vi "Read_Write_Trav_position.vi"(2 "Matched Configurations In":T1[](array[typedef]) {"Static Drive Configuration"."Indexer Mode  (FSA)" items=["Incremental", "Absolute"]; "Static Drive Configuration"."Buffer at Stop (SSH)" items=["Clear buffer", "Save and Continue"]; "Static Drive Configuration"."Buffer at Limit (SSG)" items=["Clear buffer", "Save and Continue"]; "Static Drive Configuration"."RS232 Echo Control (SSA)" items=["Echo ON", "Echo OFF"]; "Static Drive Configuration"."Reference edge of Home (OSH)" items=["CW", "CCW"]; "Static Drive Configuration"."Encoder Z for Home (OSD)" items=["Don't use", "Enable"]; "Static Drive Configuration"."Home Switch Sense (OSC)" items=["Normally Open", "Normally Closed"]; "Static Drive Configuration"."Home Position (OSB)" items=["Anywhere in Switch", "Edge of Switch"]; "Static Drive Configuration"."Limit Switch Sense (OSA)" items=["Normally Closed", "Normally Open"]; "Static Drive Configuration"."Limit Disable (LD)" items=["Both Enabled", "CW Disabled", "CCW Disabled", "Both Disabled"]; "Static Drive Configuration"."Stall Detect (FSH)" items=["Disable", "Enable"]; "Static Drive Configuration"."OP2 in Deadband (FSG)" items=["Don't Use", "ACTIVATE"]; "Static Drive Configuration"."Stop on Trigger 3 (FSF)" items=["Ignore", "STOP!"]; "Static Drive Configuration"."Activate OP1 on stall (FSE)" items=["Do not Activate", "ACTIVATE!"]; "Static Drive Configuration"."Stop on Stall (FSD)" items=["Continue", "STOP"]; "Static Drive Configuration"."Position Maintenance (FSC)" items=["Disabled", "Enabled"]; "Static Drive Configuration"."Step Mode  (FSB)" items=["Motor", "Encoder"]; "Static Drive Configuration"."Encoder Resolution (ER)" min=1 max=50000; "Static Drive Configuration"."Dead Band Window (DW)" min=0 max=999999999; "Static Drive Configuration"."Dead Band (DB)" min=0 max=999999999; "Static Drive Configuration"."Correction Gain % (CG)" items=["n/a", "12.5", "25", "37.5", "50", "62.5", "75", "87.5", "100"]; "Channel Properties"."Current Pos" format="%.2f"; "Channel Properties"."Backlash/Eng units" format="%.2f"; "Channel Properties"."Pulses/rev" format="%.2f"; "Channel Properties"."Pos Tolerance" format="%.2f"; "Channel Properties"."Pulses/unit" format="%.2f"; "Channel Properties"."Acc. Min" format="%.2f"; "Channel Properties"."Acc. Max" format="%.2f"; "Channel Properties"."Vel. Min" format="%.2f"; "Channel Properties"."Vel. Max" format="%.2f"; "Channel Properties"."Acc. Default" format="%.2f"; "Channel Properties"."Vel. Default" format="%.2f"}, 3 "Mode":T4(ring), 4 "Traverse Name":string="EnFlo Tunnel") -> (0 "Matched Configurations Out":T1[](array[typedef]) {"Static Drive Configuration"."Indexer Mode  (FSA)" items=["Incremental", "Absolute"]; "Static Drive Configuration"."Buffer at Stop (SSH)" items=["Clear buffer", "Save and Continue"]; "Static Drive Configuration"."Buffer at Limit (SSG)" items=["Clear buffer", "Save and Continue"]; "Static Drive Configuration"."RS232 Echo Control (SSA)" items=["Echo ON", "Echo OFF"]; "Static Drive Configuration"."Reference edge of Home (OSH)" items=["CW", "CCW"]; "Static Drive Configuration"."Encoder Z for Home (OSD)" items=["Don't use", "Enable"]; "Static Drive Configuration"."Home Switch Sense (OSC)" items=["Normally Open", "Normally Closed"]; "Static Drive Configuration"."Home Position (OSB)" items=["Anywhere in Switch", "Edge of Switch"]; "Static Drive Configuration"."Limit Switch Sense (OSA)" items=["Normally Closed", "Normally Open"]; "Static Drive Configuration"."Limit Disable (LD)" items=["Both Enabled", "CW Disabled", "CCW Disabled", "Both Disabled"]; "Static Drive Configuration"."Stall Detect (FSH)" items=["Disable", "Enable"]; "Static Drive Configuration"."OP2 in Deadband (FSG)" items=["Don't Use", "ACTIVATE"]; "Static Drive Configuration"."Stop on Trigger 3 (FSF)" items=["Ignore", "STOP!"]; "Static Drive Configuration"."Activate OP1 on stall (FSE)" items=["Do not Activate", "ACTIVATE!"]; "Static Drive Configuration"."Stop on Stall (FSD)" items=["Continue", "STOP"]; "Static Drive Configuration"."Position Maintenance (FSC)" items=["Disabled", "Enabled"]; "Static Drive Configuration"."Step Mode  (FSB)" items=["Motor", "Encoder"]; "Static Drive Configuration"."Encoder Resolution (ER)" min=1 max=50000; "Static Drive Configuration"."Dead Band Window (DW)" min=0 max=999999999; "Static Drive Configuration"."Dead Band (DB)" min=0 max=999999999; "Static Drive Configuration"."Correction Gain % (CG)" items=["n/a", "12.5", "25", "37.5", "50", "62.5", "75", "87.5", "100"]; "Channel Properties"."Current Pos" format="%.2f"; "Channel Properties"."Backlash/Eng units" format="%.2f"; "Channel Properties"."Pulses/rev" format="%.2f"; "Channel Properties"."Pos Tolerance" format="%.2f"; "Channel Properties"."Pulses/unit" format="%.2f"; "Channel Properties"."Acc. Min" format="%.2f"; "Channel Properties"."Acc. Max" format="%.2f"; "Channel Properties"."Vel. Min" format="%.2f"; "Channel Properties"."Vel. Max" format="%.2f"; "Channel Properties"."Acc. Default" format="%.2f"; "Channel Properties"."Vel. Default" format="%.2f"})   [LabVIEW 2011]
uses:
  AxisConfigCluster.ctl
  DriveProperties.ctl
  DriveStaticConfig.ctl
  Anemometry/Anemometry Sub Vis/Globals/Constants_global.vi
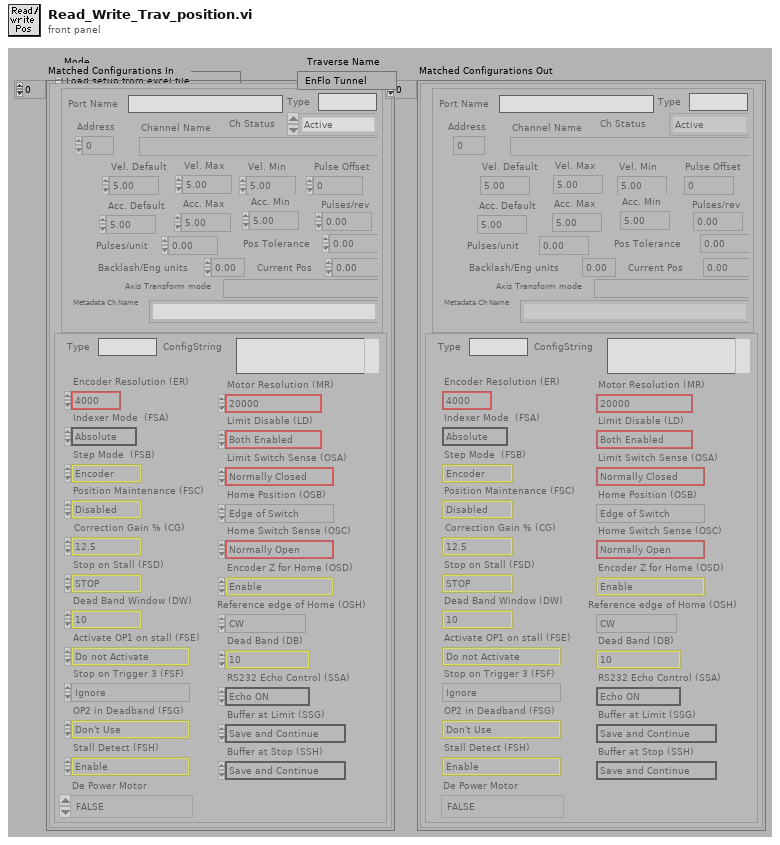
[diagram p1: front panel]
types:
  T1 = typedef "AxisConfigCluster.ctl" = cluster{"Channel Properties":T2, "Static Drive Configuration":T3}
  T2 = typedef "DriveProperties.ctl" = cluster{"Channel Name":string, "Vel. Default":dbl, "Acc. Default":dbl, "Vel. Max":dbl, "Vel. Min":dbl, "Acc. Max":dbl, "Acc. Min":dbl, "Pulses/unit":dbl, "Address":u8, "Pulse Offset":i32, "Pos Tolerance":dbl, "Pulses/rev":dbl, "Backlash/Eng units":dbl, "Current Pos":dbl, "Ch Status":enum16{"Active", "Offline", "Simulate"}, "Port Name":string, "Axis Transform mode":string, "Metadata Ch Name":string, "Type":string}
  T3 = typedef "DriveStaticConfig.ctl" = cluster{"Correction Gain % (CG)":u16, "Dead Band (DB)":i32, "Dead Band Window (DW)":i32, "Encoder Resolution (ER)":i32, "Step Mode  (FSB)":u16, "Position Maintenance (FSC)":u16, "Stop on Stall (FSD)":u16, "Activate OP1 on stall (FSE)":u16, "Stop on Trigger 3 (FSF)":u16, "OP2 in Deadband (FSG)":u16, "Stall Detect (FSH)":u16, "Limit Disable (LD)":u16, "Motor Resolution (MR)":enum16{"200", "400", "1000", "2000", "4000", "5000", "10000", "12800", "18000", "20000", "21600", "25000", "25400", "25600", "36000", "50000", "278528", "425984", "507904", "614400", "655360", "819200", "1024000"}, "Limit Switch Sense (OSA)":u16, "Home Position (OSB)":u16, "Home Switch Sense (OSC)":u16, "Encoder Z for Home (OSD)":u16, "Reference edge of Home (OSH)":u16, "RS232 Echo Control (SSA)":u16, "Buffer at Limit (SSG)":u16, "Buffer at Stop (SSH)":u16, "Indexer Mode  (FSA)":u16, "Type":string, "ConfigString":string, "De Power Motor":enum16{"TRUE", "FALSE"}}
  T4 = enum16{"Load setup from excel file", "Save setup to excel file"}
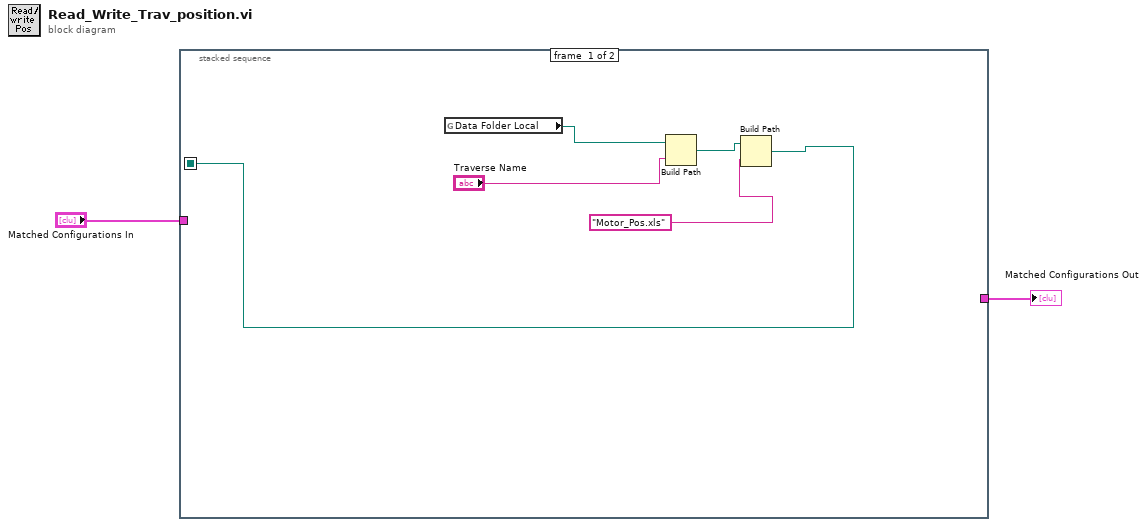
[diagram p0: block diagram]
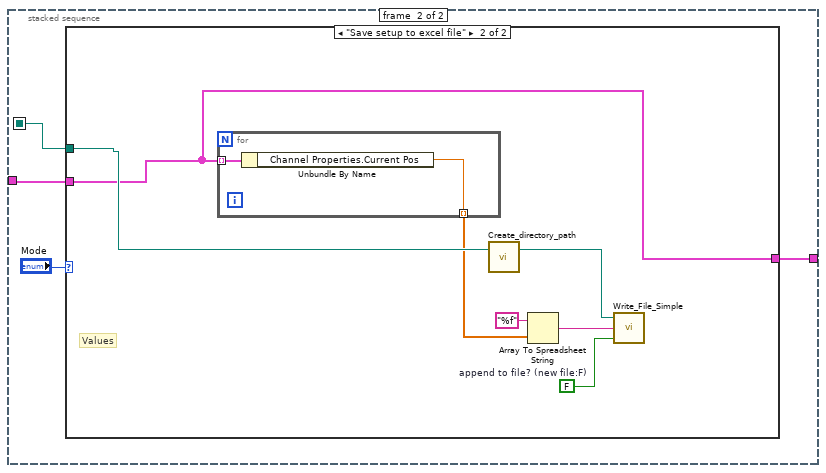
[diagram p2: hidden frame]
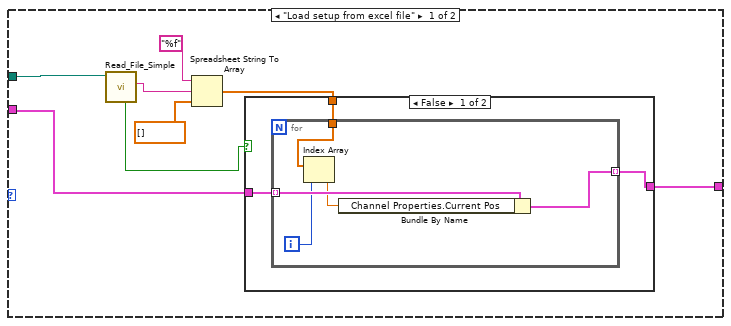
[diagram p3: hidden frame]
diagram:
  n1 = stacked-sequence {
    seq-local: [w4 _] -> [_ w10]
    tunnel: "Matched Configurations In" -> [_ w9]
    tunnel: [_ w8] -> w1
    frame #0 {
      n2 = global read "Constants_global.vi" "Data Folder Local"() -> (w5:path)
      n3 = Build Path(base path=w5, name or relative path="Traverse Name") -> (appended path=w3:path)
      n4 = Build Path(base path=w3, name or relative path="Motor_Pos.xls" ("Substring")) -> (appended path=w4:path)
    }
    frame #1 {
      n5 = case shown="\"Save setup to excel file\"" "Mode" {
        tunnel: w10 -> [w19 w31]
        tunnel: w9 -> [w18 w29]
        tunnel: [w17 w29] -> w8
        frame "Load setup from excel file" {
          n6 = call "Read_File_Simple.vi"("Filename"=w19) -> ("Error?"=w12:bool, "string"=w14:string)  [unwired: 2 in, 6 out]
          n7 = Spreadsheet String To Array(format string="%f", spreadsheet string=w14, array type (2D Dbl)=dbl[] []) -> (array=w13:dbl[])  [unwired: 1 out]
          n8 = case shown="False" w12 {
            tunnel: w18 -> [w22 w28]
            tunnel: [w21 w28] -> w17
            tunnel: w13 -> [w20 _]
            frame False {
              n9 = for {
                tunnel: w22 -> [w27] mode=indexing
                tunnel: [w26] -> w21 mode=indexing
                tunnel: w20 -> [w25]
                i -> [w24]
                n10 = Index Array(array=w25, index=w24) -> (element=w23:dbl)
                n11 = Bundle By Name(cluster=w27, "Channel Properties.Current Pos"=w23) -> (w26:T1)
              }
            }
            frame True {
            }
          }
        }
        frame "Save setup to excel file" {
          w33 = FALSE  # append to file? (new file:F)
          # "Values"
          n12 = for {
            tunnel: w29 -> [w37] mode=indexing
            tunnel: [w36] -> w30 mode=indexing
            n13 = Unbundle By Name(w37) -> ("Channel Properties.Current Pos"=w36:dbl)
          }
          n14 = call "Create_directory_path.vi"("Path name"=w31) -> ("Path name Out"=w35:path)  [unwired: 1 in, 1 out]
          n15 = Array To Spreadsheet String(array=w30, 3:"%f" ("format string")) -> (spreadsheet string=w34:string)  [unwired: 1 out]
          n16 = call "Write_File_Simple.vi"("append to file? (new file:F)"=w33, "character string"=w34, "file path"=w35) -> ()  [unwired: 2 out]
        }
      }
    }
  }
  "Matched Configurations Out" <- w1
